vi "CRC.vi"(11 "字符串":string="\u0001\u0003\u0010\u0001\u0000\u0001") -> (1 "CRC":string, 3 "连接的字符串":string)   [LabVIEW 2017]
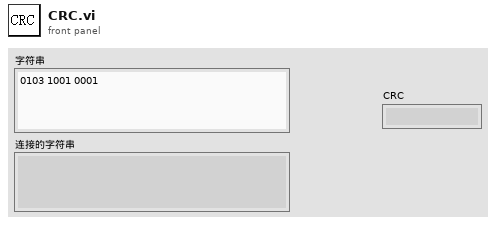
[diagram p1: front panel]
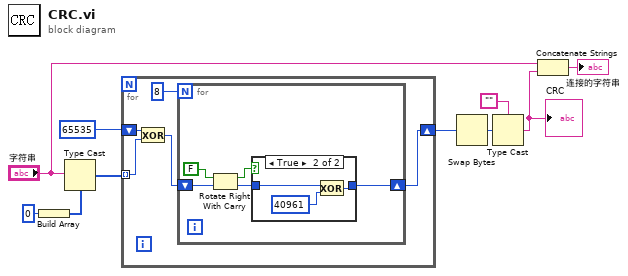
[diagram p0: block diagram]
diagram:
  n1 = Build Array(u8 0) -> (w5:u8[])
  n2 = Type Cast(type=w5, x="字符串") -> (*(type *) &x=w6:u8[])
  n3 = for {
    shift-right: [w12] -> w3
    shift-left: u16 65535 ("y") -> [w15]
    tunnel: w6 -> [w11] mode=indexing
    n4 = Exclusive Or(1:w11, 2:w15) -> (0:w13:u16)
    n5 = for {
      N: 8 -> [_]
      shift-right: [w17] -> w12
      shift-left: w13 -> [w20]
      n6 = Rotate Right With Carry(2:w20, 3:FALSE ("carry")) -> (0:w16:u16, 1:w18:bool)
      n7 = case shown="True" w18 {
        tunnel: w16 -> [w21 w24]
        tunnel: [w21 w22] -> w17
        frame False {
        }
        frame True {
          n8 = Exclusive Or(1:u16 40961 ("y"), 2:w24) -> (0:w22:u16)
        }
      }
    }
  }
  n9 = Swap Bytes(anything=w3) -> (byte swapped=w8:u16)
  n10 = Type Cast(type="", x=w8) -> (*(type *) &x=w9:string)
  "CRC" <- w9
  n11 = Concatenate Strings("字符串", w9) -> (→"连接的字符串":string)
